vi "Read Experiment Configuration.vi"(8 "error in (no error)":errorcluster, 11 "AFM Control":refnum<class "AFM Control.lvclass">) -> (0 "error out":errorcluster, 2 "Experiment Description":T1={"User"="", "Device"="", "Device Path"=path "", "Device Description"="", "Experiment Path"=path "", "Experiment Description"="", "Instrument"=enum."MNK"}, 3 "AFM Control out":refnum<class "AFM Control.lvclass">)   [LabVIEW 2016, in "AFM Control.lvclass"]
uses:
  AFM Control.lvclass
  Typedefs/Experiment Description--cluster.ctl
  Typedefs/Instrument--enum.ctl
  AFM Control.lvclass/AFM Control.ctl
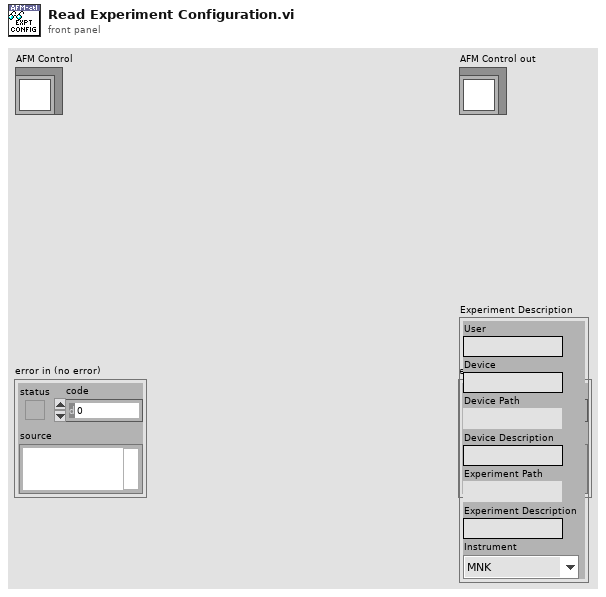
[diagram p1: front panel]
types:
  T1 = typedef "AFM Control.lvclass/Experiment Description--cluster.ctl" = cluster{"User":string, "Device":string, "Device Path":path, "Device Description":string, "Experiment Path":path, "Experiment Description":string, "Instrument":T2}
  T2 = typedef "AFM Control.lvclass/Instrument--enum.ctl" = enum16{"PPMS", "PPMS2", "MFP3D", "CYPHER", "THz1", "THz2", "MNK", "CF900", "JEOL", "AGILENT", "EBL"}
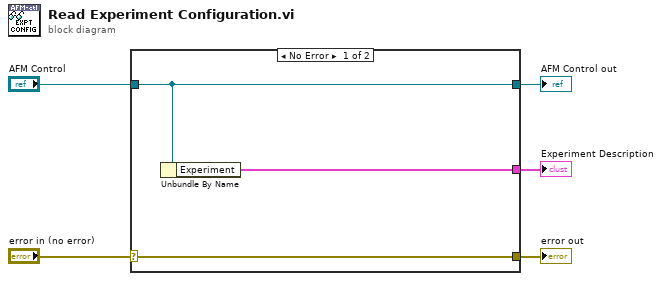
[diagram p0: block diagram]
diagram:
  n1 = case shown="No Error" "error in (no error)" {
    selector: "error in (no error)" -> [w8 w9]
    tunnel: [w8 w9] -> w4
    tunnel: [w7 w10] -> w2
    tunnel: "AFM Control" -> [w7 w10]
    tunnel: [w6 _] -> w1
    frame No Error {
      n2 = Unbundle By Name(w7) -> ("Experiment"=w6:T1)
    }
    frame Error {
    }
  }
  "error out" <- w4
  "AFM Control out" <- w2
  "Experiment Description" <- w1
